vi "Set Map Size.vi"(8 "error in (no error)":errorcluster, 10 "Map Size":i32, 11 "Game in":refnum<class "Game.lvclass">) -> (0 "error out":errorcluster, 3 "Game out":refnum<class "Game.lvclass">)   [LabVIEW 2020, in "SquareBattle.lvlib" / "Game.lvclass"]
uses:
  Game.lvclass
  Game.lvclass/Game.ctl
  Map/Map.lvclass
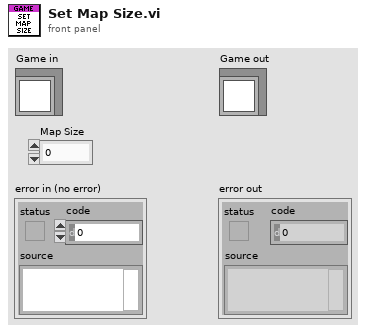
[diagram p1: front panel]
types:
  T1 = typedef "SquareBattle.lvlib/Position.ctl" = cluster{"Row":i32, "Col":i32}
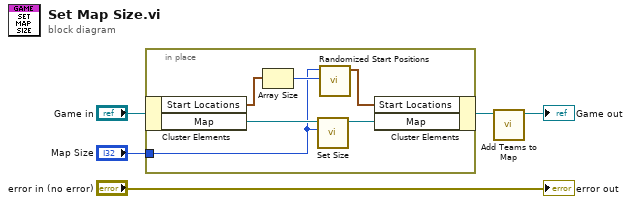
[diagram p0: block diagram]
diagram:
  n1 = in-place {
    in-place-border: "Map Size" -> [w7]
    n2 = in-place-cluster #1("Game in") -> ("Start Locations"=w9:T1[], "Map"=w11:refnum<class "Map.lvclass">)
    n3 = Array Size(array=w9) -> (size(s)=w8:i32)
    n4 = call "Set Size.vi"("Size"=w7, "Map in"=w11) -> ("Map out"=w10:refnum<class "Map.lvclass">)  [unwired: 8 in, 1 out]
    n5 = call "Randomized Start Positions.vi"("Player Count"=w8, "Size"=w7) -> ("Positions"=w6:T1[])  [unwired: 9 in]
    n6 = in-place-cluster #1("Start Locations"=w6, "Map"=w10) -> (w2:refnum<class "Game.lvclass">)
  }
  n7 = call "Add Teams to Map.vi"("Game in"=w2) -> ("Game out"=→"Game out":refnum<class "Game.lvclass">)  [unwired: 10 in]
  "error out" <- "error in (no error)"
